vi "Eliminate Wrong Target.vi"(1 "Particle Reports (Pixels)":T1(array[cluster]) {"Orientation" format="%.2f"; "Dimensions"."Height" format="%.2f"; "Dimensions"."Width" format="%.2f"; "Center of Mass"."Y" format="%.2f"; "Center of Mass"."X" format="%.2f"; "Bounding Rect"."Bottom" format="%.2f"; "Bounding Rect"."Right" format="%.2f"; "Bounding Rect"."Top" format="%.2f"; "Bounding Rect"."Left" format="%.2f"; "Number of Holes" format="%.2f"; "Area" format="%.2f"}) -> (0 "Target Particle Reports (Pixels)":T1(array[cluster]))   [LabVIEW 2016]
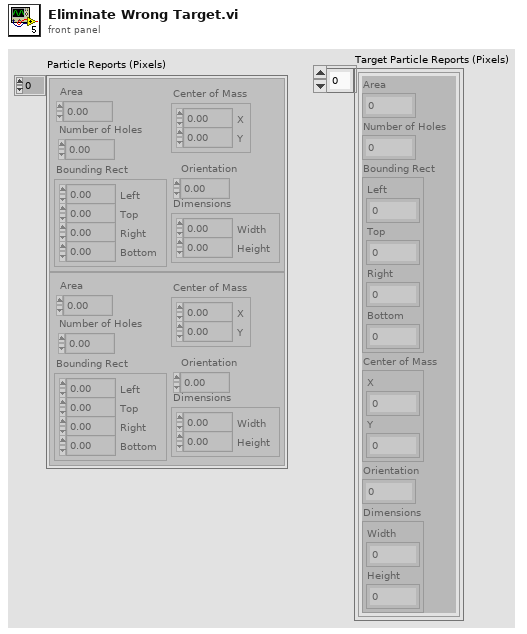
[diagram p1: front panel]
types:
  T1 = cluster{"Area":dbl, "Number of Holes":dbl, "Bounding Rect":cluster{"Left":dbl, "Top":dbl, "Right":dbl, "Bottom":dbl}, "Center of Mass":cluster{"X":dbl, "Y":dbl}, "Orientation":dbl, "Dimensions":cluster{"Width":dbl, "Height":dbl}}[]
  T2 = cluster{"Area":dbl, "Number of Holes":dbl, "Bounding Rect":cluster{"Left":dbl, "Top":dbl, "Right":dbl, "Bottom":dbl}, "Center of Mass":cluster{"X":dbl, "Y":dbl}, "Orientation":dbl, "Dimensions":cluster{"Width":dbl, "Height":dbl}}
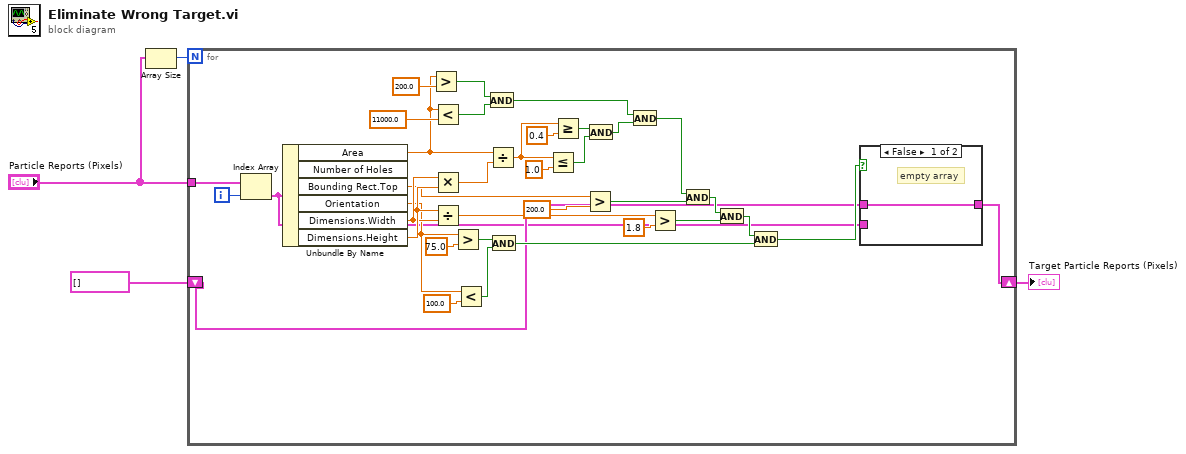
[diagram p0: block diagram]
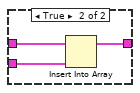
[diagram p2: hidden frame]
diagram:
  n1 = Array Size(array="Particle Reports (Pixels)") -> (size(s)=w4:i32)
  n2 = for {
    N: w4 -> [_]
    tunnel: "Particle Reports (Pixels)" -> [w16]
    shift-right: [w10] -> w1
    shift-left: T1 [] ("Particle Reports (Pixels) 2") -> [w12]
    i -> [w17]
    n3 = Index Array(array=w16, index=w17) -> (element=w11:T2)
    n4 = Unbundle By Name(w11) -> ("Area"=w5:dbl, "Bounding Rect.Top"=w14:dbl, "Orientation"=w26:dbl, "Dimensions.Width"=w35:dbl, "Dimensions.Height"=w36:dbl)  [unwired: 1 out]
    n5 = Greater?(x=w5, y=200.0) -> (0:w7:bool)
    n6 = Less?(x=w5, y=11000.0) -> (x < y?=w9:bool)
    n7 = Multiply(x=w35, y=w36) -> (x*y=w38:dbl)
    n8 = Divide(x=w36, y=w35) -> (x/y=w34:dbl)
    n9 = Greater?(x=w26, y=75.0) -> (0:w28:bool)
    n10 = Less?(x=w26, y=100.0) -> (x < y?=w27:bool)
    n11 = And(x=w7, y=w9) -> (x .and. y?=w6:bool)
    n12 = Divide(x=w5, y=w38) -> (x/y=w37:dbl)
    n13 = And(x=w28, y=w27) -> (x .and. y?=w24:bool)
    n14 = Less Or Equal?(x=w37, y=1.0) -> (x <= y?=w39:bool)
    n15 = Greater Or Equal?(x=w37, y=0.4) -> (x >= y?=w40:bool)
    n16 = Greater?(x=w14, y=200.0) -> (0:w31:bool)
    n17 = And(x=w40, y=w39) -> (x .and. y?=w33:bool)
    n18 = And(x=w6, y=w33) -> (x .and. y?=w32:bool)
    n19 = Greater?(x=w34, y=1.8) -> (0:w29:bool)
    n20 = And(x=w32, y=w31) -> (x .and. y?=w30:bool)
    n21 = And(x=w30, y=w29) -> (x .and. y?=w25:bool)
    n22 = And(x=w25, y=w24) -> (x .and. y?=w13:bool)
    n23 = case shown="False" w13 {
      tunnel: w12 -> [w41 w44]
      tunnel: w11 -> [_ w43]
      tunnel: [w41 w42] -> w10
      frame False {
        # "empty array"
      }
      frame True {
        n24 = Insert Into Array(array=w44, new element=w43) -> (w42:T1)  [unwired: 1 in]
      }
    }
  }
  "Target Particle Reports (Pixels)" <- w1
